vi "Get Self Queue.vi"(11 "Addresses in":refnum<class "Addresses.lvclass">) -> (2 "Self Queue":refnum<data-value>)   [LabVIEW 2021, in "jettl.lvlib" / "Addresses.lvlib" / "Addresses.lvclass"]
uses:
  Addresses.lvclass
  Msg Strategy/Msg Strategy.lvclass
  Addresses.lvclass/Addresses.ctl
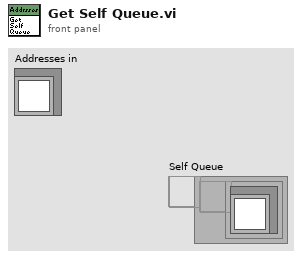
[diagram p1: front panel]
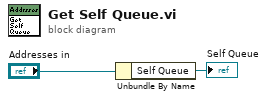
[diagram p0: block diagram]
diagram:
  n1 = Unbundle By Name("Addresses in") -> ("Self Queue"=→"Self Queue":refnum<data-value>)
